vi "Time.vi"(8 "error in (no error)":errorcluster, 10 "Control In":T1, 11 "C4 Dispense in":refnum<class "Iterative Dispense.lvclass">) -> (0 "error out":errorcluster, 1 "Timing Data":i32[](array[numeric]), 2 "Control Out":T1, 3 "C4 Dispense out":refnum<class "Iterative Dispense.lvclass">)   [LabVIEW 2019, in "Iterative Dispense.lvclass"]
uses:
  Iterative Dispense.lvclass
  Controller/Controllers.ctl
  Controller/I-O/I-O.lvclass
  Controller/Dispenser/Dispenser.lvclass
  C:/Program Files (x86)/Aerotech/A3200/LabVIEW/2010/Bin/Aerotech.A3200.dll
  Program Files (x86)/Aerotech/A3200/LabVIEW/2010/Bin/Aerotech.A3200.dll
  Iterative Dispense.lvclass/Iterative Dispense.ctl
  Controller/Motion/A3200/A3200.lvclass
  Controller/Controller.lvclass
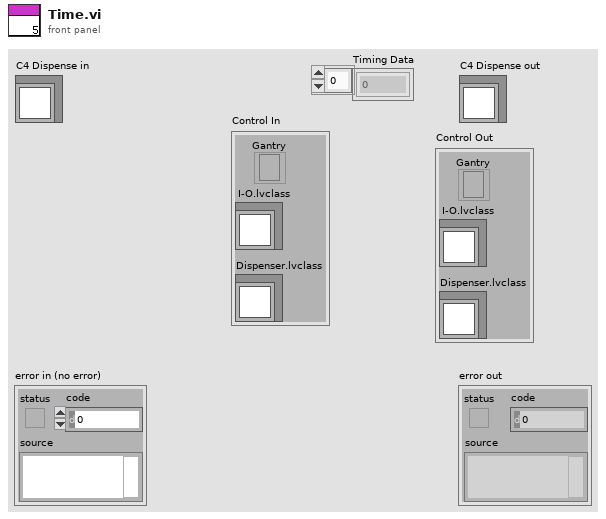
[diagram p1: front panel]
types:
  T1 = typedef "Controller.lvclass/Controllers.ctl" = cluster{"I-O.lvclass":refnum<class "I-O.lvclass">, "Dispenser.lvclass":refnum<class "Dispenser.lvclass">, "Gantry":refnum<k24>}
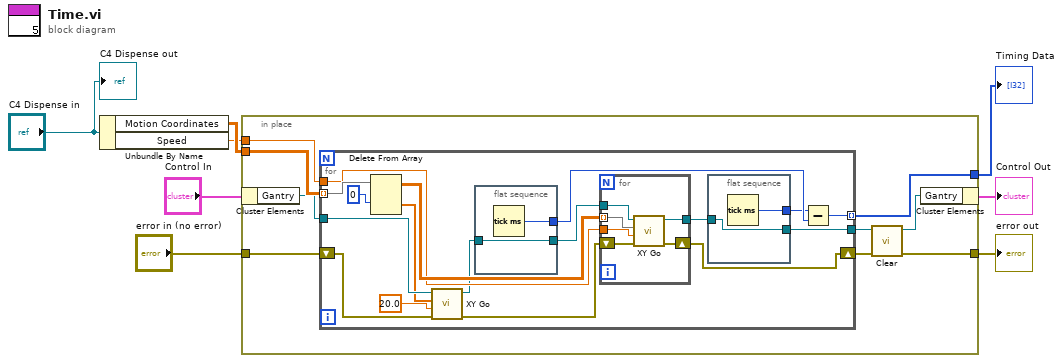
[diagram p0: block diagram]
diagram:
  n1 = Unbundle By Name("C4 Dispense in") -> ("Motion Coordinates"=w8:dbl[][][], "Speed"=w3:dbl)
  n2 = in-place {
    in-place-border: w8 -> [w17]
    in-place-border: [w16] -> w7
    in-place-border: w3 -> [w15]
    in-place-border: "error in (no error)" -> [w11]
    in-place-border: [w9] -> w1
    n3 = in-place-cluster #1("Control In") -> ("Gantry"=w14:refnum<k24>)
    n4 = for {
      tunnel: [w32] -> w13
      tunnel: [w30] -> w16 mode=indexing
      tunnel: w17 -> [w27] mode=indexing
      tunnel: w15 -> [w26]
      tunnel: w14 -> [w24]
      shift-right: [w18] -> w10
      shift-left: w11 -> [w20]
      n5 = Delete From Array(array=w27, index (row)=0) -> (deleted portion=w22:dbl[], array with subset deleted=w29:dbl[][])  [unwired: 2 in]
      n6 = call "XY Go.vi"("error in (no error)"=w20, "Speed"=20.0, "XY"=w22, "Gantry In"=w24) -> ("error out"=w19:errorcluster, "Gantry Out"=w21:refnum<k24>)  [unwired: 6 in]
      n7 = flat-sequence {
        tunnel: [w38] -> w34
        tunnel: [w37] -> w25
        tunnel: w21 -> [w37]
        frame #0 {
          n8 = Tick Count (ms)() -> (millisecond timer value=w38:u32)
        }
      }
      n9 = for {
        tunnel: [w41] -> w33
        tunnel: w29 -> [w44] mode=indexing
        tunnel: w26 -> [w43]
        tunnel: w25 -> [w42]
        shift-right: [w39] -> w18
        shift-left: w19 -> [w40]
        n10 = call "XY Go.vi"("error in (no error)"=w40, "Speed"=w43, "XY"=w44, "Gantry In"=w42) -> ("error out"=w39:errorcluster, "Gantry Out"=w41:refnum<k24>)  [unwired: 6 in]
      }
      n11 = flat-sequence {
        tunnel: w33 -> [w36]
        tunnel: [w36] -> w32
        tunnel: [w35] -> w31
        frame #0 {
          n12 = Tick Count (ms)() -> (millisecond timer value=w35:u32)
        }
      }
      n13 = Subtract(x=w31, y=w34) -> (x-y=w30:u32)
    }
    n14 = call "Clear.vi"("error in (no error)"=w10, "Gantry In"=w13) -> ("error out"=w9:errorcluster, "Gantry Out"=w12:refnum<k24>)  [unwired: 8 in]
    n15 = in-place-cluster #1("Gantry"=w12) -> (→"Control Out":T1)
  }
  "error out" <- w1
  "Timing Data" <- w7
  "C4 Dispense out" <- "C4 Dispense in"
